vi "Save Image.vi"(8 "error in (no error)":errorcluster, 10 "Shift":u32, 11 "CCDCamera in":refnum<class "CCDCamera.lvclass">) -> (0 "error out":errorcluster, 3 "CCDCamera out":refnum<class "CCDCamera.lvclass">)   [LabVIEW 2018, in "CCDCamera.lvclass"]
uses:
  CCDCamera.lvclass
  <userlib>/gfitsio/cfitsio-bitpix.ctl
  CCDCamera.lvclass/CCDCamera.ctl
  <userlib>/gfitsio/gfitsio-write-image-subset-i16-2d.vi
  <userlib>/gfitsio/gfitsio.lvlib
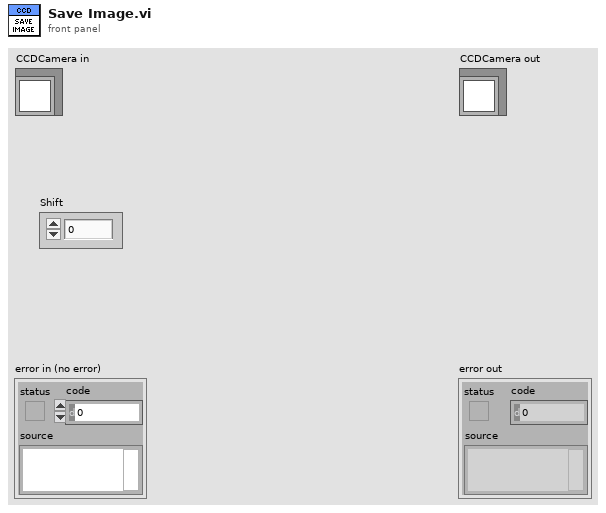
[diagram p1: front panel]
types:
  T1 = enum16{"open", "open or create", "create or replace", "create", "open (read only)"}
  T2 = enum16{"open", "open or create", "create", "create or replace"}
  T3 = typedef "gfitsio.lvlib/cfitsio-bitpix.ctl" = i32
  T4 = typedef "gfitsio.lvlib/gfitsio-refnum.ctl" = refnum<k1>
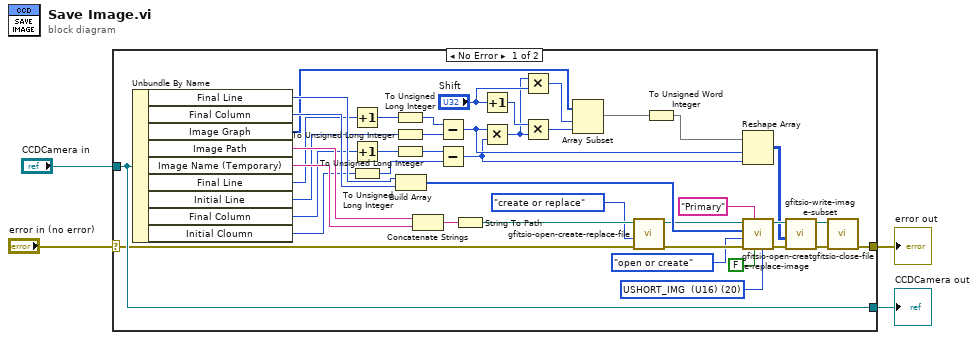
[diagram p0: block diagram]
diagram:
  n1 = case shown="No Error" "error in (no error)" {
    selector: "error in (no error)" -> [w41 w48]
    tunnel: [w40 w48] -> w2
    tunnel: [w46 w47] -> w3
    tunnel: "CCDCamera in" -> [w46 w47]
    frame No Error {
      w34 = T3 20 items=["<invalid type>"=0, "BYTE_IMG  (U8)"=8, "SHORT_IMG  (I16)"=16, "USHORT_IMG  (U16)"=20, "LONG_IMG  (I32)"=32, "ULONG_IMG  (U32)"=40, "FLOAT_IMG  (SGL)"=-32, "DOUBLE_IMG  (DBL)"=-64] ("image data type")
      n2 = Unbundle By Name(w46) -> ("Final Line"=w44:u16, "Final Column"=w45:u16, "Image Graph"=w25:u16[], "Image Path"=w33:string, "Image Name (Temporary)"=w32:string, "Final Line"=w10:u16, "Initial Line"=w14:u16, "Final Column"=w8:u16, "Initial Cloumn"=w17:u16)
      n3 = Increment(x=w10) -> (x+1=w11:u16)
      n4 = Increment(x=w8) -> (x+1=w9:u16)
      n5 = To Unsigned Long Integer(number=w17) -> (unsigned 32bit integer=w16:u32)
      n6 = To Unsigned Long Integer(number=w11) -> (unsigned 32bit integer=w12:u32)
      n7 = To Unsigned Long Integer(number=w14) -> (unsigned 32bit integer=w13:u32)
      n8 = To Unsigned Long Integer(number=w9) -> (unsigned 32bit integer=w15:u32)
      n9 = Build Array(w44, w45) -> (w39:u16[])
      n10 = Concatenate Strings(w33, w32) -> (w31:string)
      n11 = Subtract(x=w12, y=w13) -> (x-y=w24:u32)
      n12 = Subtract(x=w15, y=w16) -> (x-y=w23:u32)
      n13 = String To Path(string=w31) -> (path=w30:path)
      n14 = Increment(x="Shift") -> (x+1=w20:u32)
      n15 = Multiply(x=w24, y=w23) -> (x*y=w19:u32)
      n16 = Multiply(x=w19, y="Shift") -> (x*y=w22:u32)
      n17 = Multiply(x=w20, y=w19) -> (x*y=w18:u32)
      n18 = Array Subset(array=w25, index=w22, length=w18) -> (w6:u16[])
      n19 = call <userlib>:"gfitsio-open-create-replace-file.vi"("error in (no error)"=w41, "function (open)"=T1."create or replace", "file path (dialog if empty)"=w30) -> ("error out"=w43:errorcluster, "gfits refnum"=w38:T4)  [unwired: 6 in, 1 out]
      n20 = To Unsigned Word Integer(number=w6) -> (unsigned 16bit integer=w5:u16[])
      n21 = Reshape Array(w5, w24, w23) -> (w7:u16[][])
      n22 = call <userlib>:"gfitsio-open-create-replace-image.vi"("image data type"=w34, "advisory dialog? (display:T)"=FALSE, "hdu name (dialog if empty)"="Primary" ("prompt"), "error in (no error)"=w43, "function (open or create)"=T2."open or create", "naxes"=w39, "gfits refnum"=w38) -> ("error out"=w42:errorcluster, "dup gfits refnum"=w37:T4)  [unwired: 2 in, 1 out]
      n23 = call-poly <userlib>:"gfitsio-write-image-subset.vi"("error in (no error)"=w42, "data"=w7, "gfits refnum"=w37) -> ("error out"=w26:errorcluster, "dup gfits refnum"=w27:T4)  [unwired: 7 in]
      n24 = call <userlib>:"gfitsio-close-file.vi"("error in (no error)"=w26, "gfits refnum"=w27) -> ("error out"=w40:errorcluster)  [unwired: 8 in, 1 out]
    }
    frame Error {
    }
  }
  "error out" <- w2
  "CCDCamera out" <- w3
